vi "数据标识判定.vi"(8 "通讯故障":bool, 9 "量程下限":dbl, 10 "量程上限":dbl, 11 "测量值":sgl) -> (3 "数据标识":string)   [LabVIEW 2016, in "斯坦道多参数.lvlib"]
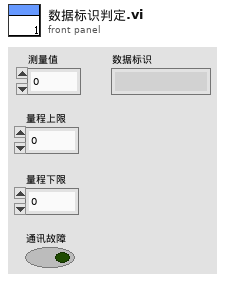
[diagram p1: front panel]
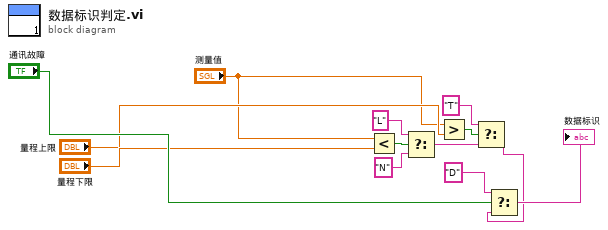
[diagram p0: block diagram]
diagram:
  n1 = Less?(x="测量值", y="量程下限") -> (x < y?=w6:bool)
  n2 = Select(t="L", s=w6, f="N") -> (s? t:f=w9:string)
  n3 = Greater?(x="测量值", y="量程上限") -> (0:w4:bool)
  n4 = Select(t="T", s=w4, f=w9) -> (s? t:f=w12:string)
  n5 = Select(t="D", s="通讯故障", f=w12) -> (s? t:f=→"数据标识":string)
